vi "Coord window-Shortcut menu selection handler.vi"(10 "Shortcut menu itemTag":string) -> (0 "error out":errorcluster)   [LabVIEW 2020]
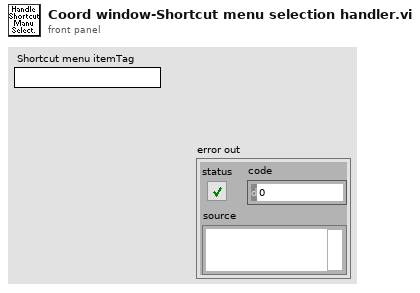
[diagram p1: front panel]
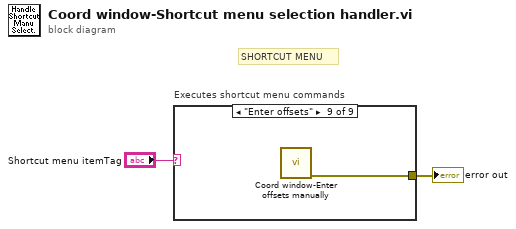
[diagram p0: block diagram]
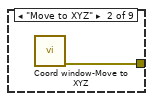
[diagram p3: hidden frame]
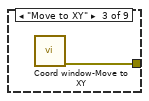
[diagram p4: hidden frame]
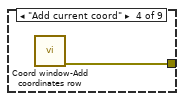
[diagram p5: hidden frame]
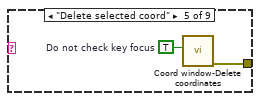
[diagram p6: hidden frame]
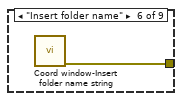
[diagram p7: hidden frame]
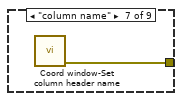
[diagram p8: hidden frame]
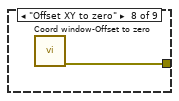
[diagram p9: hidden frame]
diagram:
  # "SHORTCUT MENU"
  n1 = case "Executes shortcut menu commands" shown="\"Enter offsets\"" "Shortcut menu itemTag" {
    tunnel: [_ w3 w4 w5 w7 w8 w9 w10 w11] -> w1
    frame Default {
    }
    frame "Move to XYZ" {
      n2 = call "Coord window-Move to XYZ.vi"() -> ("error out"=w3:errorcluster)  [unwired: 11 in]
    }
    frame "Move to XY" {
      n3 = call "Coord window-Move to XY.vi"() -> ("error out"=w4:errorcluster)  [unwired: 11 in]
    }
    frame "Add current coord" {
      n4 = call "Coord window-Add coordinates row.vi"() -> ("error out"=w5:errorcluster)  [unwired: 11 in]
    }
    frame "Delete selected coord" {
      w6 = TRUE  # Do not check key focus
      n5 = call "Coord window-Delete coordinates.vi"("Do not check key focus"=w6) -> ("error out"=w7:errorcluster)  [unwired: 10 in]
    }
    frame "Insert folder name" {
      n6 = call "Coord window-Insert folder name string.vi"() -> ("error out"=w8:errorcluster)  [unwired: 11 in]
    }
    frame "column name" {
      n7 = call "Coord window-Set column header name.vi"() -> ("error out"=w9:errorcluster)  [unwired: 11 in]
    }
    frame "Offset XY to zero" {
      n8 = call "Coord window-Offset to zero.vi"() -> ("error out"=w10:errorcluster)  [unwired: 11 in]
    }
    frame "Enter offsets" {
      n9 = call "Coord window-Enter offsets manually.vi"() -> ("error out"=w11:errorcluster)  [unwired: 11 in]
    }
  }
  "error out" <- w1
